vi "ServoGetPosMax.vi"(0 "error in (no error)":errorcluster, 2 "index":i32, 3 "Device In":i32) -> (7 "error out":errorcluster, 9 "posmax_out":dbl, 10 "Device Out":i32)   [LabVIEW 2012]
uses:
  phidget21.dll
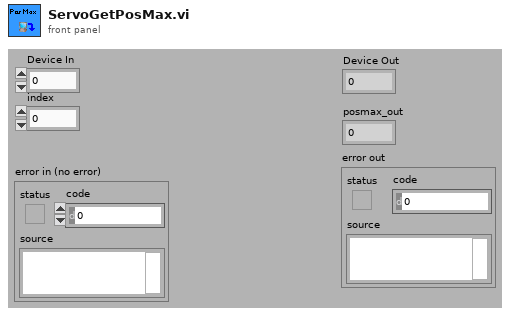
[diagram p1: front panel]
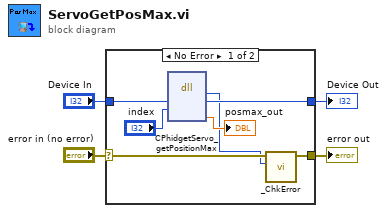
[diagram p0: block diagram]
diagram:
  n1 = case shown="No Error" "error in (no error)" {
    selector: "error in (no error)" -> [w7 w13]
    tunnel: [w6 w13] -> w3
    tunnel: "Device In" -> [w9 w12]
    tunnel: [w8 w12] -> w1
    frame No Error {
      n2 = dll-call lib="phidget21.*" fn="CPhidgetServo_getPositionMax"("phid"=w9, "index"="index") -> (w5:i32, "phid"=w8:i32, "posmax_out"=→"posmax_out":dbl)  [unwired: 5 in, 2 out]
      n3 = call "_ChkError.vi"("Return Code"=w5, "error in (no error)"=w7) -> ("error out"=w6:errorcluster)  [unwired: 9 in]
    }
    frame Error {
    }
  }
  "error out" <- w3
  "Device Out" <- w1
